vi "Gui_SetupProcessing.vi"(8 "error in (no error)":errorcluster, 11 "Variant":variant) -> (0 "error out":errorcluster caption="sortie d'erreur", 3 "Variant out":variant)   [LabVIEW 2020]
doc: "This VI setup the PROCESSING parameters.\n\n1. The PROCESSING parameters are passed by a Variant as input.\n2. Init the controls with the previous values.\n3. Wait for the user events, and update controls accordingly.\n4. When OK is pushed, return an updated Variant as output.\n5. When CANCEL is pushed, restore previous values."
uses:
  controls/PROCESSING_Inputs.ctl
  controls/SEQUENCE_Inputs.ctl
  controls/EXCIT_Inputs.ctl
  controls/DATA_Inputs.ctl
  controls/TIMING_Inputs.ctl
  controls/TRAPPING_Inputs.ctl
panel:
  out "PROCESSING Inputs 2":T1={"Reference Mass"=300.0939, "Cyclotron Freq"=255.727, "Magnetron Freq"=0.001} {"Magnetron Freq" format="%.5g"; "Cyclotron Freq" format="%.5g"; "Reference Mass" format="%.5g"}
  in  "CANCEL":bool
  in  "SEQUENCE Inputs":T2={"EXCIT Inputs"={"Number of Excitations"=1, "Script Text"="", "Table of Waveforms"=[]}, "DATA Inputs"={"Record Length"=8192, "Sample Rate"=4.0, "Data Type"=0, "Vertical Range"=0.0, "Acquisition Duration"=100000.0}, "TIMING Inputs"={"Number of Acquisitions "=1, "Number of Accumulations"=1, "Table of Waveforms"=[], "Script Text"=""}, "PROCESSING Inputs"={"Reference Mass"=300.0939, "Cyclotron Freq"=255.727, "Magnetron Freq"=0.001}, "TRAPPING Inputs"={"Number of Channels"=4, "Init Values"=[2.0, 5.0, 5.0, 2.0], "Opening Values"=[0.0, 0.0, 0.0, 0.0], "Trapping Values"=[2.0, 5.0, 5.0, 2.0], "Emptying Values"=[-5.0, -5.0, -5.0, -5.0], "Adiabatic ON"=FALSE, "Adiabatic Duration"=0, "Adiabatic Waveforms"=["Adiabatic_None_2_2_2000.bin", "Adiabatic_Ramp_5_0_2000.bin", "Adiabatic_DoubleRamp_5_0_2000.bin", "Adiabatic_RC_2_0_2000.bin"], "Ions Refill ON"=FALSE, "Number of Ions Refills"=4}} {"TRAPPING Inputs"."Number of Ions Refills" min=1 max=1000; "TRAPPING Inputs"."Trapping Values" min=-10.0 max=10.0; "TRAPPING Inputs"."Init Values" min=-10.0 max=10.0; "TRAPPING Inputs"."Emptying Values" min=-10.0 max=10.0; "TRAPPING Inputs"."Opening Values" min=-10.0 max=10.0; "PROCESSING Inputs"."Magnetron Freq" format="%.5g"; "PROCESSING Inputs"."Cyclotron Freq" format="%.5g"; "PROCESSING Inputs"."Reference Mass" format="%.5g"; "TIMING Inputs"."Number of Accumulations" min=0 max=50 step=1; "TIMING Inputs"."Number of Acquisitions" min=1 max=10 step=1; "DATA Inputs"."Vertical Range" items=["0.2"=0.2, "0.4"=0.4, "1"=1.0, "2"=2.0, "4"=4.0, "10"=10.0]; "DATA Inputs"."Data Type" items=["I16", "DBL"]; "DATA Inputs"."Sample Rate" items=["1 MHz"=1000000.0, "2 MHz"=2000000.0, "5 MHz"=5000000.0, "10 MHz"=10000000.0, "20 MHz"=20000000.0, "25 MHz"=25000000.0, "50 MHz"=50000000.0, "100 MHz"=100000000.0]; "EXCIT Inputs"."Number of Excitations" min=1 max=10}
  in  "PROCESSING Inputs":T1={"Reference Mass"=300.0939, "Cyclotron Freq"=255.727, "Magnetron Freq"=0.001} caption="DATA Inputs" {"Magnetron Freq" format="%.5g"; "Cyclotron Freq" format="%.5g"; "Reference Mass" format="%.5g"}
  in  "OK":bool
  # "GO_out"
  # "Gout"
  # "GI_in"
  # "Gin"
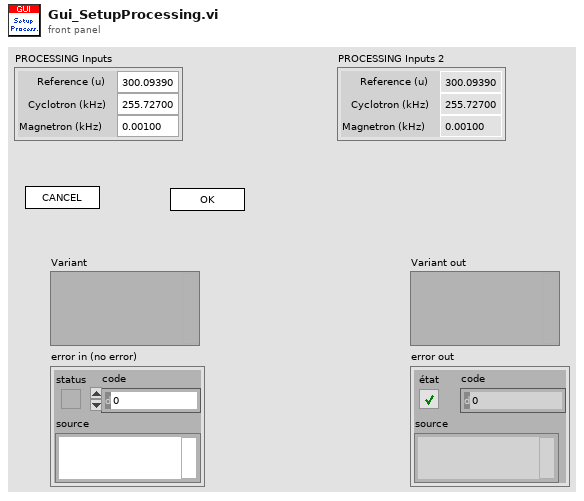
[diagram p1: front panel]
types:
  T1 = typedef "PROCESSING_Inputs.ctl" = cluster{"Reference Mass":dbl, "Cyclotron Freq":dbl, "Magnetron Freq":dbl}
  T2 = typedef "SEQUENCE_Inputs.ctl" = cluster{"EXCIT Inputs":T3, "DATA Inputs":T4, "TIMING Inputs":T5, "PROCESSING Inputs":T1, "TRAPPING Inputs":T6}
  T3 = typedef "EXCIT_Inputs.ctl" = cluster{"Number of Excitations":i32, "Script Text":string, "Table of Waveforms":string[]}
  T4 = typedef "DATA_Inputs.ctl" = cluster{"Record Length":i32, "Sample Rate":dbl, "Data Type":u8, "Vertical Range":dbl, "Acquisition Duration":dbl}
  T5 = typedef "TIMING_Inputs.ctl" = cluster{"Number of Acquisitions ":i16, "Number of Accumulations":i16, "Table of Waveforms":string[], "Script Text":string}
  T6 = typedef "TRAPPING_Inputs.ctl" = cluster{"Number of Channels":i32, "Init Values":dbl[], "Opening Values":dbl[], "Trapping Values":dbl[], "Emptying Values":dbl[], "Adiabatic ON":bool, "Adiabatic Duration":i32, "Adiabatic Waveforms":string[], "Ions Refill ON":bool, "Number of Ions Refills":i32}
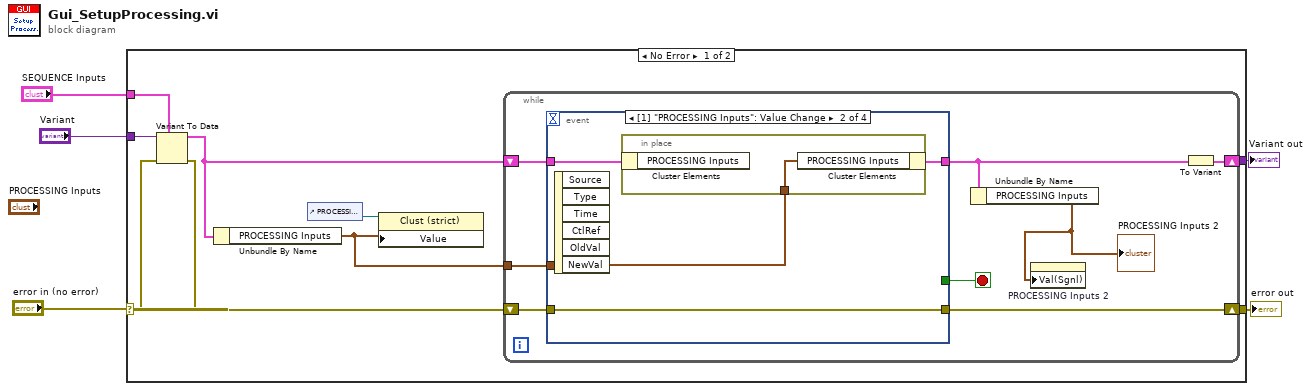
[diagram p0: block diagram]
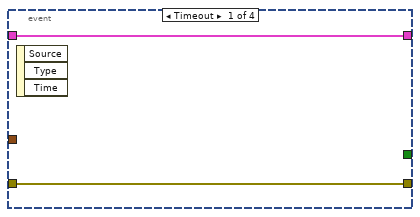
[diagram p2: hidden frame]
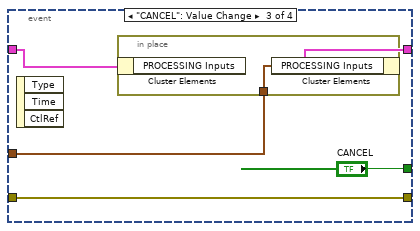
[diagram p3: hidden frame]
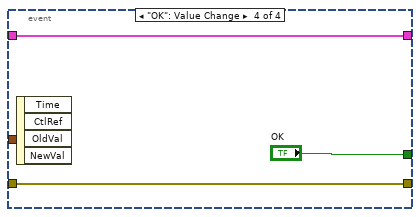
[diagram p4: hidden frame]
diagram:
  n1 = case shown="No Error" "error in (no error)" {
    selector: "error in (no error)" -> [w7 w40]
    tunnel: [w15 w40] -> w4
    tunnel: "Variant" -> [w14 w39]
    tunnel: [w11 w39] -> w2
    tunnel: "SEQUENCE Inputs" -> [w10 _]
    frame No Error {
      n2 = Variant To Data(error in=w7, type=w10, Variant=w14) -> (data=w13:T2, error out=w6:errorcluster)
      n3 = Unbundle By Name(w13) -> ("PROCESSING Inputs"=w9:T1)
      n4 = control-ref of="PROCESSING Inputs"() -> (w8:refnum<vi>)
      n5 = property class="Clust (strict)"(reference=w8, "Value"=w9) -> ()  [unwired: 1 in, 2 out]
      n6 = while {
        shift-right: [w19] -> w15
        shift-left: w6 -> [w20]
        shift-right: [w17] -> w12
        shift-left: w13 -> [w22]
        tunnel: w9 -> [w18]
        stop <- w21 stop-if-true
        n7 = event shown="[1] \"PROCESSING Inputs\": Value Change" {
          selector: _ -> [_ _ _ _]
          dyn-events: _ -> [_ _ _ _]
          timeout: _ -> [_ _ _ _]
          tunnel: w22 -> [w24 w28 w32 w36]
          tunnel: [w24 w27 w31 w36] -> w17
          tunnel: [_ _ "CANCEL" "OK"] -> w21
          tunnel: w20 -> [w23 w26 w33 w37]
          tunnel: [w23 w26 w33 w37] -> w19
          tunnel: w18 -> [_ _ w30 _]
          event Timeout {
            n8 = event-data() -> ()  [unwired: 1 in, 3 out]
          }
          event Value Change {
            n9 = event-data() -> ("NewVal"=w25:T1)  [unwired: 1 in, 5 out]
            n10 = in-place {
              in-place-border: w25 -> [w29]
              n11 = in-place-cluster #1(w28) -> ()  [unwired: 1 out]
              n12 = in-place-cluster #1("PROCESSING Inputs"=w29) -> (w27:T2)
            }
          }
          event "CANCEL": Value Change {
            n13 = event-data() -> ()  [unwired: 1 in, 3 out]
            n14 = in-place {
              in-place-border: w30 -> [w35]
              n15 = in-place-cluster #2(w32) -> ()  [unwired: 1 out]
              n16 = in-place-cluster #2("PROCESSING Inputs"=w35) -> (w31:T2)
            }
          }
          event "OK": Value Change {
            n17 = event-data() -> ()  [unwired: 1 in, 4 out]
          }
        }
        n18 = Unbundle By Name(w17) -> ("PROCESSING Inputs"=w16:T1)
        "PROCESSING Inputs 2" <- w16
        n19 = property on="PROCESSING Inputs 2" class="Clust (strict)"("Val(Sgnl)"=w16) -> ()  [unwired: 2 in, 2 out]
      }
      n20 = To Variant(anything=w12) -> (Variant=w11:variant)
    }
    frame Error {
    }
  }
  "error out" <- w4
  "Variant out" <- w2
